vi "_Save Config File.vi"(4 "Sample List":string[][](table), 5 "AcqMethod":T1[](array[typedef]) {"ScanType" format="%#.6g"; "Mass Range"."Res" items=["High/High", "Medium/Medium", "Low/Low", "High/Medium", "High/Low", "Medium/High", "Medium/Low", "Low/High", "Low/Medium"]}, 6 "GUI Method":T8={"Lenses"=[], "Mass Ranges"=[], "Acquire"=FALSE, "MCA"=FALSE, "Q1DC EN"=FALSE, "Q1 POL"=FALSE, "Q3 POL"=FALSE, "Q1 RF  EN"=FALSE, "Averaging"=FALSE, "Log Scale"=FALSE, "CPS"=FALSE, "Unit"=FALSE, "Data Path"=path "", "Run Mode"=enum."MRM (Q1/Q2)", "Fixed Mass (amu)"=1.0, "Q3DC EN"=FALSE, "Q3 RF  EN"=FALSE, "Negative"=FALSE} {"Mass Ranges"."Res" items=["High/High", "Medium/Medium", "Low/Low", "High/Medium", "High/Low", "Medium/High", "Medium/Low", "Low/High", "Low/Medium"]}, 7 "File Type (config)":T11, 8 "advisory dialog? (display:T)":bool=TRUE, 9 "Cal/Res":dbl[][](array[numeric]), 10 "Configuration":T6, 11 "start path  (Not A Path)":path=path "") -> (0 "error":bool, 2 "Config Out":T6, 3 "new file path":path)   [LabVIEW 2012]
doc: "Reads and plots data previously stored with the Write to Text File.vi example. The VI reads one line at a time, splits off the first (timestamp) column from the subsequent data columns, then converts the data to numbers and plots them. See sprdsht.llb for more information on spreadsheet format."
uses:
  Type/_File Type.ctl
  Type/_RT Instrument 2.ctl
  Type/_RT Configuration 2.ctl
  Type/_GUI Method.ctl
  Type/_Lens Property.ctl
  Type/_Mass Range Property.ctl
  Type/_Mass Range Parameters.ctl
  Type/_RT Res Type.ctl
  Type/_Run Mode.ctl
  Type/_XML Expt.ctl
  Type/_XML Lens.ctl
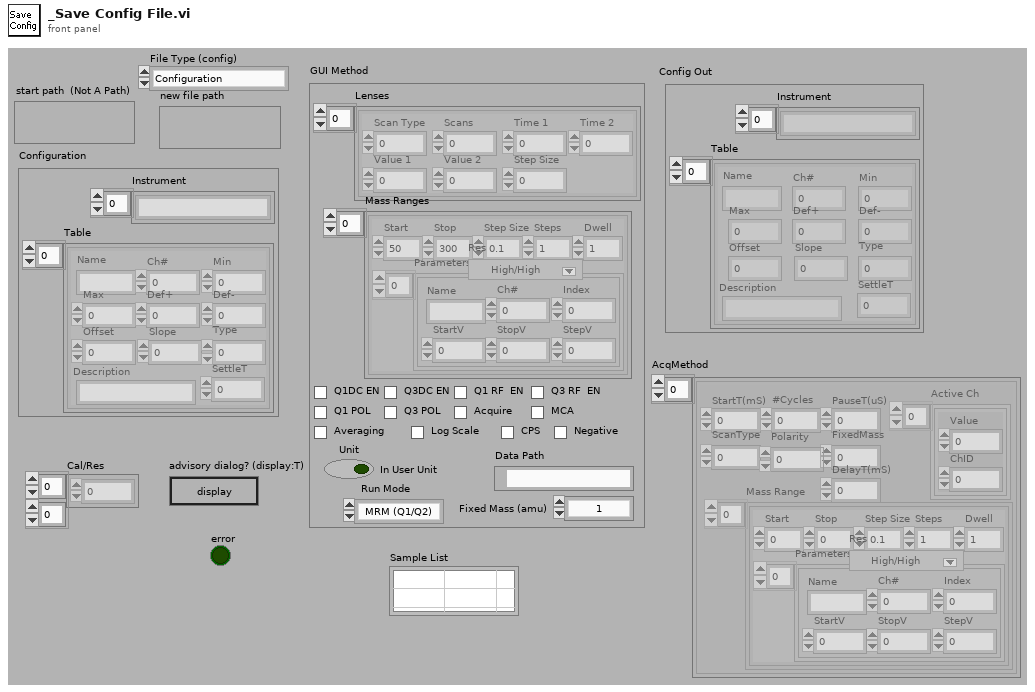
[diagram p1: front panel]
types:
  T1 = typedef "_XML Expt.ctl" = cluster{"StartT(mS)":i32, "#Cycles":i32, "PauseT(uS)":i32, "ScanType":i32, "Polarity":u8, "FixedMass":dbl, "DelayT(mS)":i32, "Active Ch":T2[], "Mass Range":T3[]}
  T2 = typedef "_XML Lens.ctl" = cluster{"Value":dbl, "ChID":u8}
  T3 = typedef "_Mass Range Property.ctl" = cluster{"Start":dbl, "Stop":dbl, "Step Size":dbl, "Steps":i32, "Dwell":dbl, "Parameters":T4[], "Res":T5}
  T4 = typedef "_Mass Range Parameters.ctl" = cluster{"Name":string, "Ch#":u8, "StartV":dbl, "StopV":dbl, "StepV":dbl, "Index":u8}
  T5 = typedef "_RT Res Type.ctl" = u16
  T6 = typedef "_RT Instrument 2.ctl" = cluster{"Table":T7[], "Instrument":string[]}
  T7 = typedef "_RT Configuration 2.ctl" = cluster{"Name":string, "Ch#":u8, "Min":dbl, "Max":dbl, "Def+":dbl, "Def-":dbl, "Offset":dbl, "Slope":dbl, "Type":u8, "Description":string, "SettleT":dbl}
  T8 = typedef "_GUI Method.ctl" = cluster{"Lenses":T9[], "Mass Ranges":T3[], "Acquire":bool, "MCA":bool, "Q1DC EN":bool, "Q1 POL":bool, "Q3 POL":bool, "Q1 RF  EN":bool, "Averaging":bool, "Log Scale":bool, "CPS":bool, "Unit":bool, "Data Path":path, "Run Mode":T10, "Fixed Mass (amu)":dbl, "Q3DC EN":bool, "Q3 RF  EN":bool, "Negative":bool}
  T9 = typedef "_Lens Property.ctl" = cluster{"Scan Type":u8, "Scans":i32, "Time 1":dbl, "Time 2":dbl, "Value 1":dbl, "Value 2":dbl, "Step Size":dbl}
  T10 = typedef "_Run Mode.ctl" = enum16{"MRM (Q1/Q2)", "Q1 Scan", "Q1 SRM", "Q2 Scan", "Q2 SRM", "Product Scan", "Precursor Scan", "Neutral Loss", "Neutral Gain"}
  T11 = typedef "_File Type.ctl" = enum16{"Configuration", "Old Configuration", "Calibration", "Resolution", "Diagnostic Method", "Old Method", "Acq Method", "Samp List"}
  T12 = enum16{"open", "replace", "create", "open or create", "replace or create", "replace or create with confirmation"}
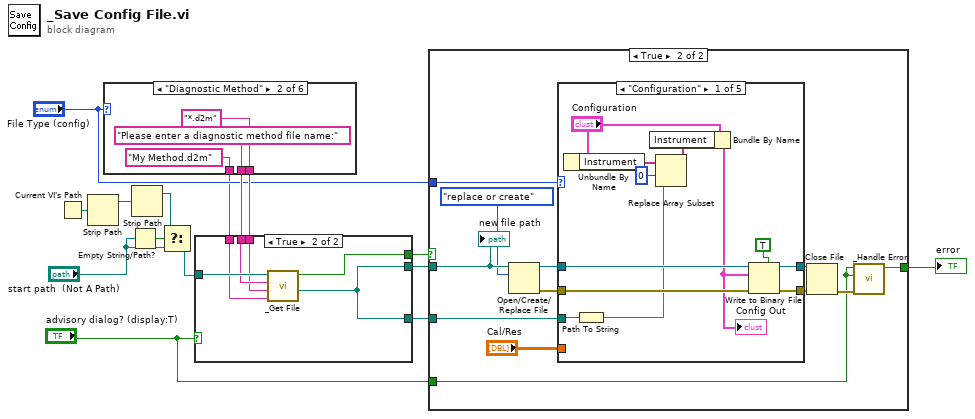
[diagram p0: block diagram]
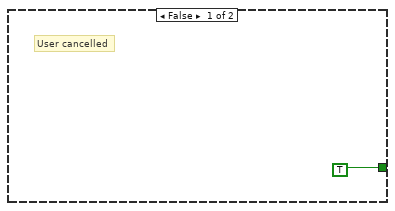
[diagram p2: hidden frame]
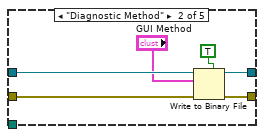
[diagram p3: hidden frame]
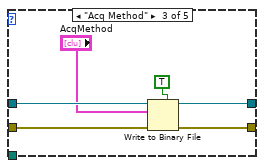
[diagram p4: hidden frame]
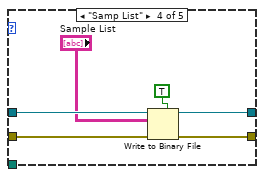
[diagram p5: hidden frame]
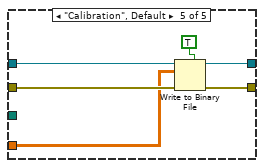
[diagram p6: hidden frame]
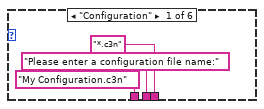
[diagram p7: hidden frame]
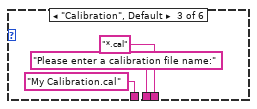
[diagram p8: hidden frame]
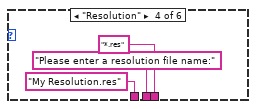
[diagram p9: hidden frame]
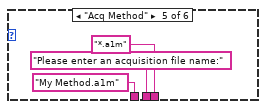
[diagram p10: hidden frame]
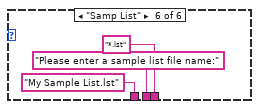
[diagram p11: hidden frame]
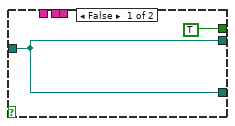
[diagram p12: hidden frame]
diagram:
  n1 = Current VI's Path() -> (path=w12:path)
  n2 = Strip Path(path=w12) -> (stripped path=w13:path)  [unwired: 1 out]
  n3 = case shown="\"Diagnostic Method\"" "File Type (config)" {
    tunnel: ["*.c3n" ("pattern (*.cfg)") "*.d2m" ("pattern (*.cfg)") "*.cal" ("pattern (*.cfg)") "*.res" ("pattern (*.cfg)") "*.a1m" ("pattern (*.cfg)") "*.lst" ("pattern (*.cfg)")] -> w7
    tunnel: ["Please enter a configuration file name:" ("prompt") "Please enter a diagnostic method file name:" ("prompt") "Please enter a calibration file name:" ("prompt") "Please enter a resolution file name:" ("prompt") "Please enter an acquisition file name:" ("prompt") "Please enter a sample list file name:" ("prompt")] -> w6
    tunnel: ["My Configuration.c3n" ("pattern (*.cfg)") "My Method.d2m" ("pattern (*.cfg)") "My Calibration.cal" ("pattern (*.cfg)") "My Resolution.res" ("pattern (*.cfg)") "My Method.a1m" ("pattern (*.cfg)") "My Sample List.lst" ("pattern (*.cfg)")] -> w1
    frame "Configuration" {
    }
    frame "Diagnostic Method" {
    }
    frame "Calibration", Default {
    }
    frame "Resolution" {
    }
    frame "Acq Method" {
    }
    frame "Samp List" {
    }
  }
  n4 = Empty String/Path?(string/path="start path  (Not A Path)") -> (empty?=w15:bool)
  n5 = Strip Path(path=w13) -> (stripped path=w11:path)  [unwired: 1 out]
  n6 = Select(t=w11, s=w15, f="start path  (Not A Path)") -> (s? t:f=w9:path)
  n7 = case shown="True" "advisory dialog? (display:T)" {
    tunnel: w6 -> [_ w40]
    tunnel: w7 -> [_ w39]
    tunnel: [w35 w38] -> w4
    tunnel: w9 -> [w35 w41]
    tunnel: [w35 w38] -> w3
    tunnel: [TRUE w37] -> w2
    tunnel: w1 -> [_ w36]
    frame False {
    }
    frame True {
      n8 = call "_Get File.vi"("default name"=w36, "extension (isd)"=w39, "prompt"=w40, "Start Path"=w41) -> ("Seleted File"=w38:path, "Succeeded"=w37:bool)  [unwired: 3 in, 1 out]
    }
  }
  n9 = case shown="True" w2 {
    tunnel: [TRUE w53] -> w10
    tunnel: "advisory dialog? (display:T)" -> [_ w51]
    tunnel: "File Type (config)" -> [_ w49]
    tunnel: w4 -> [_ w47]
    tunnel: w3 -> [_ w44]
    frame False {
      # "User cancelled"
    }
    frame True {
      n10 = Open/Create/Replace File(file path (use dialog)=w44, operation (0:open)=T12."replace or create") -> (refnum out=w46:refnum<file>, error out=w45:errorcluster)  [unwired: 4 in, 1 out]
      n11 = case shown="\"Configuration\"" w49 {
        tunnel: [w65 w68 w75 w81 w87] -> w52
        tunnel: w45 -> [w64 w69 w76 w82 w88]
        tunnel: w46 -> [w63 w71 w77 w83 w89]
        tunnel: [w62 w70 w74 w80 w86] -> w50
        tunnel: "Cal/Res" -> [_ _ _ _ w85]
        tunnel: w47 -> [w57 _ _ _ _]
        frame "Configuration" {
          n12 = Unbundle By Name("Configuration") -> ("Instrument"=w61:string[])
          n13 = Path To String(path=w57) -> (string=w56:string)
          n14 = Replace Array Subset(array=w61, new element=w56, index=0) -> (w59:string[])
          n15 = Bundle By Name(cluster="Configuration", "Instrument"=w59) -> (w55:T6)
          "Config Out" <- w55
          n16 = Write to Binary File(file (use dialog)=w63, data=w55, error in=w64, 5:TRUE ("header (F)")) -> (refnum out=w62:refnum<file>, error out=w65:errorcluster)  [unwired: 3 out]
        }
        frame "Diagnostic Method" {
          n17 = Write to Binary File(file (use dialog)=w71, data="GUI Method", error in=w69, 5:TRUE ("header (F)")) -> (refnum out=w70:refnum<file>, error out=w68:errorcluster)  [unwired: 3 out]
        }
        frame "Acq Method" {
          n18 = Write to Binary File(file (use dialog)=w77, data="AcqMethod", error in=w76, 5:TRUE ("header (F)")) -> (refnum out=w74:refnum<file>, error out=w75:errorcluster)  [unwired: 3 out]
        }
        frame "Samp List" {
          n19 = Write to Binary File(file (use dialog)=w83, data="Sample List", error in=w82, 5:TRUE ("header (F)")) -> (refnum out=w80:refnum<file>, error out=w81:errorcluster)  [unwired: 3 out]
        }
        frame "Calibration", Default {
          n20 = Write to Binary File(file (use dialog)=w89, data=w85, error in=w88, 5:TRUE ("header (F)")) -> (refnum out=w86:refnum<file>, error out=w87:errorcluster)  [unwired: 3 out]
        }
      }
      n21 = Close File(refnum=w50, error in=w52) -> (error out=w54:errorcluster)  [unwired: 1 out]
      n22 = call "_Handle Error.vi"("error in (no error)"=w54, "Display Warning (T)"=w51, "Display Error (T)"=w51) -> ("error?"=w53:bool)  [unwired: 4 out]
      "new file path" <- w44
    }
  }
  "error" <- w10
